vi "Add or Remove File Extension.vi"(9 "File extension with period":string, 11 "File name with or without extension":string) -> (1 "Without extension":string, 3 "With extension":string)   [LabVIEW 2020]
doc: "Given a filename and a specified extension, this VI returns the filename with the extension and without it. If the original filename does not have the file extension on it, it is added; otherwise, it is removed."
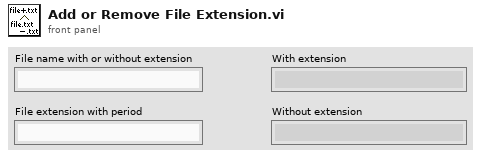
[diagram p1: front panel]
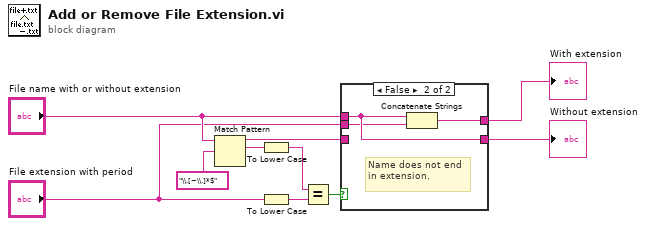
[diagram p0: block diagram]
diagram:
  n1 = Match Pattern(string="File name with or without extension", regular expression="\\.[~\\.]*$") -> (before substring=w10:string, match substring=w4:string)  [unwired: 3 out]
  n2 = To Lower Case(string=w4) -> (all lower case string=w3:string)
  n3 = To Lower Case(string="File extension with period") -> (all lower case string=w2:string)
  n4 = Equal?(x=w3, y=w2) -> (x = y?=w1:bool)
  n5 = case shown="False" w1 {
    tunnel: [w11 w15] -> w7
    tunnel: "File name with or without extension" -> [w11 w14]
    tunnel: [w12 w14] -> w6
    tunnel: w10 -> [w12 _]
    tunnel: "File extension with period" -> [_ w13]
    frame True {
      # "Name does end in extension."
    }
    frame False {
      # "Name does not end in extension."
      n6 = Concatenate Strings(w14, w13) -> (w15:string)
    }
  }
  "With extension" <- w7
  "Without extension" <- w6
